vi "List_of_running_applications.vi"(6 "error in (no error)":errorcluster) -> (0 "error out":errorcluster, 3 "TaskManager's list":string[](array[string]))   [LabVIEW 2013]
doc: "Wiebe Walstra\nwww.carya.nl\n© 2008\n\nUse freely, no warrenty."
uses:
  user32.dll
panel:
  out "Style":i32[](array[numeric]) format="%032x"
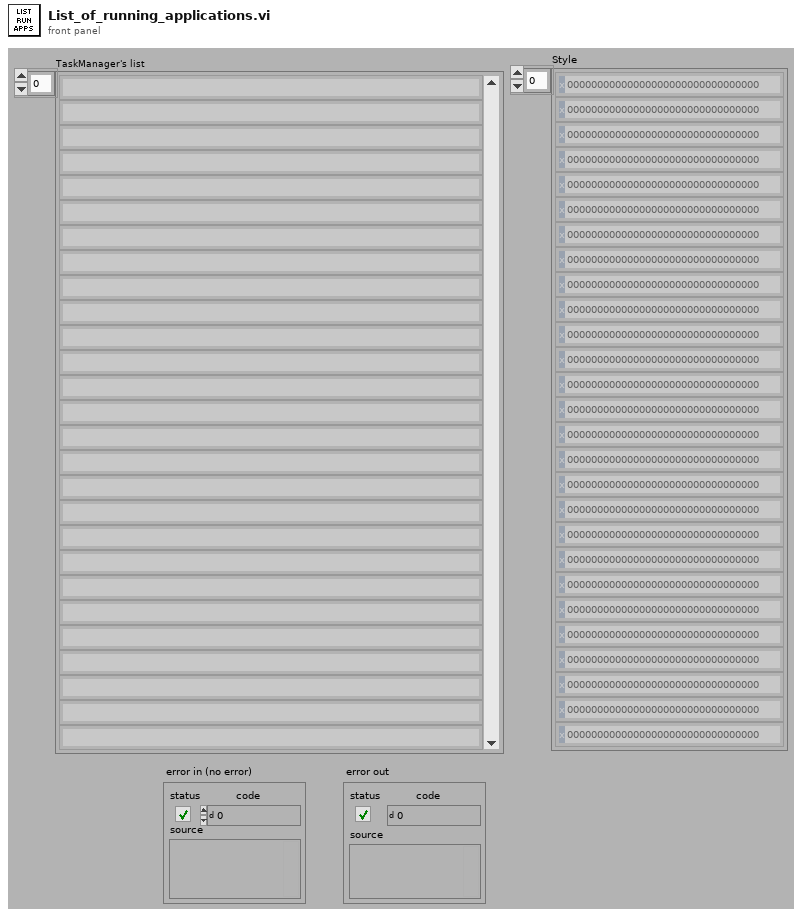
[diagram p1: front panel]
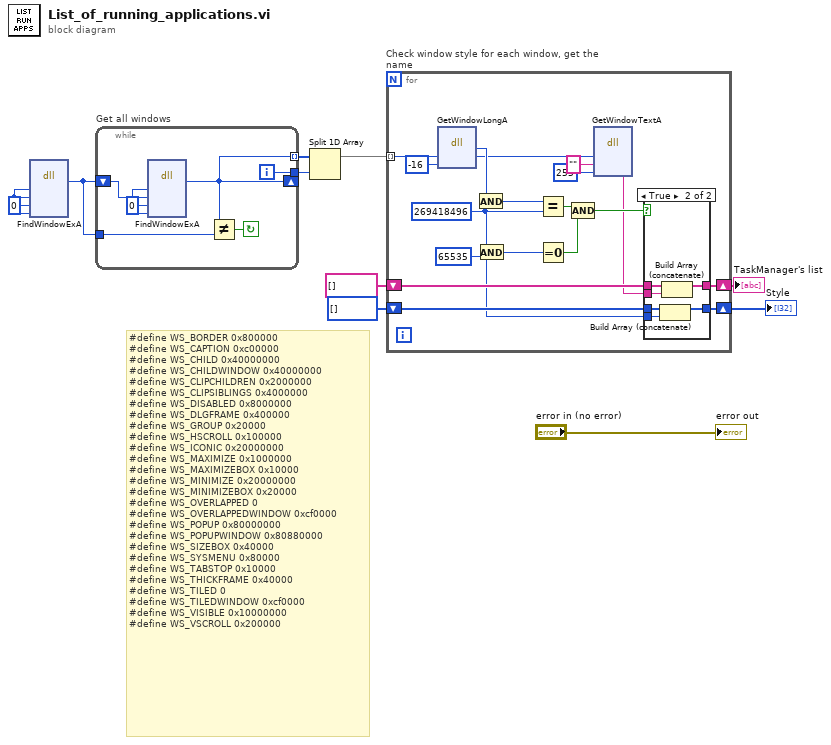
[diagram p0: block diagram]
diagram:
  w8 = 0 ("classname")
  # "#define WS_BORDER\t0x800000\n#define WS_CAPTION\t0xc00000\n#define WS_CHILD\t0x40000000\n#define WS_CHILDWINDOW\t0x40000000\n#define WS_CLIPCHILDREN 0x2000000\n#define WS_CLIPSIBLINGS 0x4000000\n#define WS_DISABLED\t0x8000000\n#define WS_DLGFRAME\t0x400000\n#define WS_GROUP\t0x20000\n#define WS_HSCROLL\t0x100000\n#define WS_ICONIC\t0x20000000\n#define WS_MAXIMIZE\t0x1000000\n#define WS_MAXIMIZEBOX\t0x10000\n#define WS_MINIMIZE\t0x20000000\n#define WS_MINIMIZEBOX\t0x20000\n#define WS_OVERLAPPED\t0\n#define WS_OVERLAPPEDWINDOW\t0xcf0000\n#define WS_POPUP\t0x80000000\n#define WS_POPUPWINDOW\t0x80880000\n#define WS_SIZEBOX\t0x40000\n#define WS_SYSMENU\t0x80000\n#define WS_TABSTOP\t0x10000\n#define WS_THICKFRAME\t0x40000\n#define WS_TILED\t0\n#define WS_TILEDWINDOW\t0xcf0000\n#define WS_VISIBLE\t0x10000000\n#define WS_VSCROLL\t0x200000"
  n1 = dll-call lib="user32.dll" fn="FindWindowExA" label="kernel32:FindWindowEx"("hWnd parent"=w8, "hWnd previous"=w8, "classname"=w8, "window name"=w8) -> ("hWnd"=w7:i32)  [unwired: 7 in, 2 out]
  n2 = while "Get all windows" {
    shift-right: [w13] -> _
    shift-left: w7 -> [w15]
    tunnel: [w13] -> w10 mode=indexing
    tunnel: [w14] -> w9
    tunnel: w7 -> [w12]
    i -> [w14]
    stop <- w11 continue-if-true
    w16 = 0 ("classname")
    n3 = dll-call lib="user32.dll" fn="FindWindowExA" label="kernel32:FindWindowEx"("hWnd parent"=w16, "hWnd previous"=w15, "classname"=w16, "window name"=w16) -> ("hWnd"=w13:i32)  [unwired: 7 in, 2 out]
    n4 = Not Equal?(x=w13, y=w12) -> (x != y?=w11:bool)
  }
  n5 = Split 1D Array(array=w10, index=w9) -> (first subarray=w6:i32[])  [unwired: 1 out]
  n6 = for "Check window style for each window, get the name" {
    tunnel: w6 -> [w18] mode=indexing
    shift-right: [w26] -> w4
    shift-left: string[] [] -> [w27]
    shift-right: [w23] -> w2
    shift-left: i32[] [] -> [w22]
    w19 = 269418496 ("y")
    n7 = dll-call lib="user32.dll" fn="GetWindowLongA" label="kernel32:FindWindowEx"("hWnd"=w18, "index"=-16) -> ("hWnd"=w21:i32, "hWnd"=w17:i32)  [unwired: 4 in, 2 out]
    n8 = And(x=w21, y=w19) -> (x .and. y?=w33:i32)
    n9 = And(x=w21, y=65535) -> (x .and. y?=w31:i32)
    n10 = Equal?(x=w33, y=w19) -> (x = y?=w28:bool)
    n11 = Equal To 0?(x=w31) -> (x = 0?=w20:bool)
    n12 = Compound Arithmetic op=AND(w28, w20) -> (w25:bool)
    n13 = dll-call lib="user32.dll" fn="GetWindowTextA" label="kernel32:FindWindowEx"("hWnd"=w17, "hWnd"="", "size"=255) -> ("hWnd"=w24:string)  [unwired: 6 in, 2 out]
    n14 = case shown="True" w25 {
      tunnel: w27 -> [w36 w42]
      tunnel: [w36 w41] -> w26
      tunnel: w24 -> [_ w40]
      tunnel: [w35 w38] -> w23
      tunnel: w22 -> [w35 w37]
      tunnel: w21 -> [_ w39]
      frame False {
      }
      frame True {
        n15 = Build Array (concatenate)(w37, w39) -> (w38:i32[])
        n16 = Build Array (concatenate)(w42, w40) -> (w41:string[])
      }
    }
  }
  "TaskManager's list" <- w4
  "Style" <- w2
  "error out" <- "error in (no error)"
